vi "obslog.vi"(4 "xmax":dbl=5.0, 6 "xmin":dbl=-5.0, 7 "FF":dbl=0.97, 8 "ymin":dbl, 9 "ymax":dbl=20.0) -> ()   [LabVIEW 2012]
uses:
  G_VEH.vi
  G_SEN.vi
  G_NAV.vi
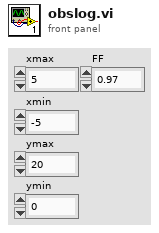
[diagram p1: front panel]
types:
  T1 = cluster{"Steer_input":dbl, "Steer_output":dbl, "VS_des":dbl, "VS_can":dbl, "heading":dbl, "auto":bool, "run":bool, "x":dbl, "y":dbl}
  T2 = cluster{"idx":i32, "x":dbl, "y":dbl, "h":dbl, "x_path":dbl}
  T3 = cluster{i16, "element":dbl, "element":dbl, "element":dbl}[]
  T4 = cluster{"GPSTime":dbl, "attitude[2]":dbl, "lcc[0]":dbl, "lcc[1]":dbl, "heading_GPS":dbl}
  T5 = cluster{i16, "element":dbl, "element":dbl, "element":dbl, "element":dbl}[]
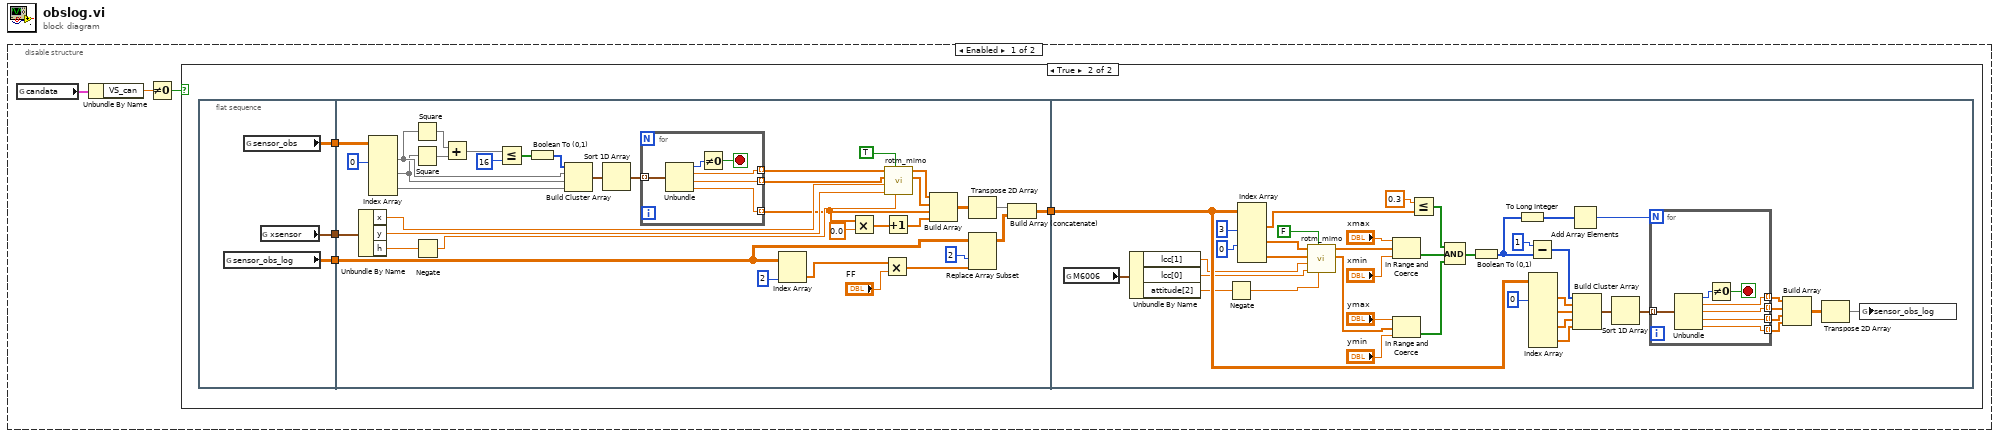
[diagram p0: block diagram]
diagram:
  n1 = disable-structure shown="Enabled" {
    frame Enabled {
      n2 = global read "G_VEH.vi" "candata"() -> (w1:T1)
      n3 = Unbundle By Name(w1) -> ("VS_can"=w2:dbl)
      n4 = Not Equal To 0?(x=w2) -> (x != 0?=w3:bool)
      n5 = case shown="True" w3 {
        frame False {
        }
        frame True {
          n6 = flat-sequence {
            tunnel: [w8] -> w7
            tunnel: [w10] -> w6
            tunnel: [w9] -> w4
            tunnel: [w30] -> w5
            tunnel: w7 -> [w17]
            tunnel: w6 -> [w16]
            tunnel: w4 -> [w15]
            tunnel: w5 -> [w94]
            frame #0 {
              n7 = global read "G_SEN.vi" "sensor_obs_log"() -> (w10:dbl[][])
              n8 = global read "G_SEN.vi" "sensor_obs"() -> (w8:dbl[][])
              n9 = global read "G_VEH.vi" "xsensor"() -> (w9:T2)
            }
            frame #1 {
              n10 = Unbundle By Name(w15) -> ("x"=w42:dbl, "y"=w43:dbl, "h"=w41:dbl)
              n11 = Index Array(array=w17, index (col) #1=0 ("disabled index (col)")) -> (element #1=w23:dbl[], element #2=w22:dbl[], element #3=w14:dbl[])  [unwired: 5 in]
              n12 = Square(x=w23) -> (x^2=w29:dbl[])
              n13 = Square(x=w22) -> (x^2=w28:dbl[])
              n14 = Negate(x=w41) -> (-x=w44:dbl)
              n15 = Add(x=w29, y=w28) -> (x+y=w27:dbl[])
              n16 = Less Or Equal?(x=w27, y=16) -> (x <= y?=w25:bool[])
              n17 = Boolean To (0,1)(Boolean=w25) -> (0, 1=w24:i16[])
              n18 = Build Cluster Array(w24, w23, w22, w14) -> (w21:T3)
              n19 = Sort 1D Array(array=w21) -> (sorted array=w20:T3)
              n20 = for {
                tunnel: w20 -> [w53] mode=indexing
                tunnel: [w50] -> w19 mode=indexing
                tunnel: [w49] -> w18 mode=indexing
                tunnel: [w48] -> w13 mode=indexing
                stop <- w51 stop-if-true
                n21 = Unbundle(w53) -> (w52:i16, "element"=w50:dbl, "element"=w49:dbl, "element"=w48:dbl)
                n22 = Not Equal To 0?(x=w52) -> (x != 0?=w51:bool)
              }
              n23 = Index Array(array=w16, index (col)=2 ("disabled index (col)")) -> (element=w35:dbl[])  [unwired: 1 in]
              n24 = Multiply(x=w13, y=0.0) -> (x*y=w38:dbl[])
              n25 = Multiply(x=w35, y="FF") -> (x*y=w33:dbl[])
              n26 = Increment(x=w38) -> (x+1=w12:dbl[])
              n27 = call "rotm_mimo.vi"("angle[rad]"=w44, "reverse"=TRUE, "y0"=w43, "x0"=w42, "y"=w18, "x"=w19) -> ("Y"=w40:dbl[], "X"=w46:dbl[])  [unwired: 2 in, 2 out]
              n28 = Build Array(w46, w40, w13, w12) -> (w11:dbl[][])
              n29 = Transpose 2D Array(2D array=w11) -> (transposed array=w32:dbl[][])
              n30 = Replace Array Subset(array=w16, new element=w33, index (col)=2 ("disabled index (col)")) -> (w31:dbl[][])  [unwired: 1 in]
              n31 = Build Array (concatenate)(w32, w31) -> (w30:dbl[][])
            }
            frame #2 {
              n32 = global read "G_NAV.vi" "M6006"() -> (w57:T4)
              n33 = Unbundle By Name(w57) -> ("lcc[1]"=w89:dbl, "lcc[0]"=w90:dbl, "attitude[2]"=w88:dbl)
              n34 = Negate(x=w88) -> (-x=w91:dbl)
              n35 = Index Array(array=w94, index (col) #1=3 ("disabled index (col)"), index (col) #2=0 ("disabled index (col)")) -> (element #1=w82:dbl[], element #2=w87:dbl[], element #3=w86:dbl[])  [unwired: 4 in]
              n36 = call "rotm_mimo.vi"("angle[rad]"=w91, "reverse"=FALSE, "y0"=w90, "x0"=w89, "y"=w86, "x"=w87) -> ("Y"=w83:dbl[], "X"=w84:dbl[])  [unwired: 2 in, 2 out]
              n37 = In Range and Coerce(upper limit="xmax", x=w84, lower limit="xmin") -> (In Range?=w80:bool[])  [unwired: 1 out]
              n38 = In Range and Coerce(upper limit="ymax", x=w83, lower limit="ymin") -> (In Range?=w78:bool[])  [unwired: 1 out]
              n39 = Less Or Equal?(x=0.3 ("thresh"), y=w82) -> (x <= y?=w79:bool[])
              n40 = Compound Arithmetic op=AND(w79, w80, w78) -> (w77:bool[])
              n41 = Boolean To (0,1)(Boolean=w77) -> (0, 1=w56:i16[])
              n42 = To Long Integer(number=w56) -> (32bit integer=w55:i32[])
              n43 = Subtract(x=i16 1, y=w56) -> (x-y=w71:i16[])
              n44 = Index Array(array=w94, index (col) #1=0 ("disabled index (col)")) -> (element #1=w69:dbl[], element #2=w68:dbl[], element #3=w67:dbl[], element #4=w59:dbl[])  [unwired: 7 in]
              n45 = Add Array Elements(numeric array=w55) -> (sum=w54:i32)
              n46 = Build Cluster Array(w71, w69, w68, w67, w59) -> (w66:T5)
              n47 = Sort 1D Array(array=w66) -> (sorted array=w65:T5)
              n48 = for {
                N: w54 -> [_]
                tunnel: w65 -> [w101] mode=indexing
                tunnel: [w98] -> w64 mode=indexing
                tunnel: [w97] -> w63 mode=indexing
                tunnel: [w96] -> w62 mode=indexing
                tunnel: [w95] -> w58 mode=indexing
                stop <- w99 stop-if-true
                n49 = Unbundle(w101) -> (w100:i16, "element"=w98:dbl, "element"=w97:dbl, "element"=w96:dbl, "element"=w95:dbl)
                n50 = Not Equal To 0?(x=w100) -> (x != 0?=w99:bool)
              }
              n51 = Build Array(w64, w63, w62, w58) -> (w61:dbl[][])
              n52 = Transpose 2D Array(2D array=w61) -> (transposed array=w60:dbl[][])
              n53 = global write "G_SEN.vi" "sensor_obs_log"(w60) -> ()
            }
          }
        }
      }
    }
    frame Disabled {
    }
  }
